vi "RemoveMean.vi"(7 "remove offset":bool, 8 "i":i32, 10 "median_in":T1, 11 "Gyro data 3DOF":sgl[](array[numeric])) -> (2 "median_out":T1)   [LabVIEW 2024]
uses:
  <vilib>/ptbypt/NI_PtbyPt.lvlib
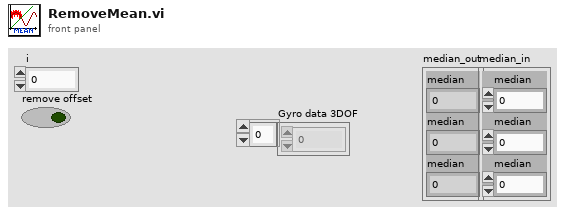
[diagram p1: front panel]
types:
  T1 = cluster{"median":dbl, "median":dbl, "median":dbl}
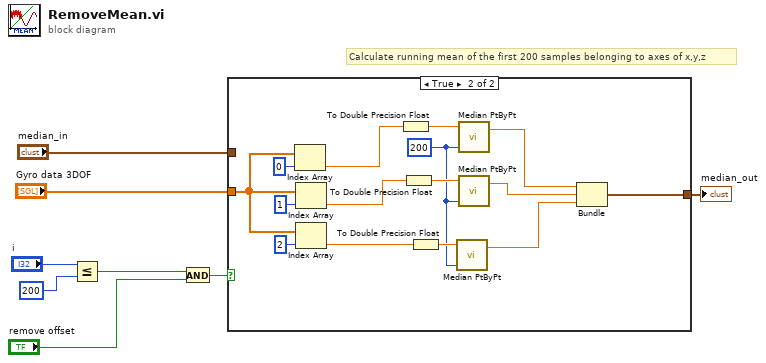
[diagram p0: block diagram]
diagram:
  # "Calculate running mean of the first 200 samples belonging to axes of x,y,z"
  n1 = Less Or Equal?(x="i", y=200) -> (x <= y?=w2:bool)
  n2 = And(x=w2, y="remove offset") -> (x .and. y?=w3:bool)
  n3 = case shown="True" w3 {
    tunnel: "Gyro data 3DOF" -> [_ w24]
    tunnel: [w9 w10] -> w5
    tunnel: "median_in" -> [w9 _]
    frame False {
    }
    frame True {
      w14 = 200 ("sample length")
      n4 = Index Array "Index Array"(array=w24, index=0) -> (element=w20:sgl)
      n5 = Index Array(array=w24, index=1) -> (element=w18:sgl)
      n6 = Index Array(array=w24, index=2) -> (element=w16:sgl)
      n7 = To Double Precision Float(number=w20) -> (double precision float=w19:dbl)
      n8 = To Double Precision Float(number=w18) -> (double precision float=w17:dbl)
      n9 = To Double Precision Float(number=w16) -> (double precision float=w15:dbl)
      n10 = call <vilib>:"Median PtByPt.vi"("sample length"=w14, "x"=w15) -> ("median"=w11:dbl)  [unwired: 2 in, 1 out]
      n11 = call <vilib>:"Median PtByPt.vi"("sample length"=w14, "x"=w19) -> ("median"=w13:dbl)  [unwired: 2 in, 1 out]
      n12 = call <vilib>:"Median PtByPt.vi"("sample length"=w14, "x"=w17) -> ("median"=w12:dbl)  [unwired: 2 in, 1 out]
      n13 = Bundle("median"=w13, "median"=w12, "median"=w11) -> (w10:T1)  [unwired: 1 in]
    }
  }
  "median_out" <- w5
